vi "List Installed Packages.vi"(8 "error in":errorcluster) -> (0 "error out":errorcluster, 2 "installed packages":string[][](table))   [LabVIEW 2014, in "NIPM_API.lvlib"]
doc: "Returns a list of all installed packages, including hidden infrastructure packages.\n\nThis list is equivalent to the list of packages in the Installed tab in NI Package Manager, with \"Settings»General»Show full version numbers and infrastructure packages\" checkbox enabled.\n\nOUTPUT(s)\n<B>Installed packages</B>: Outputs a list of installed packages"
uses:
  NIPM_API.lvlib
panel:
  out "cmd standard output":string
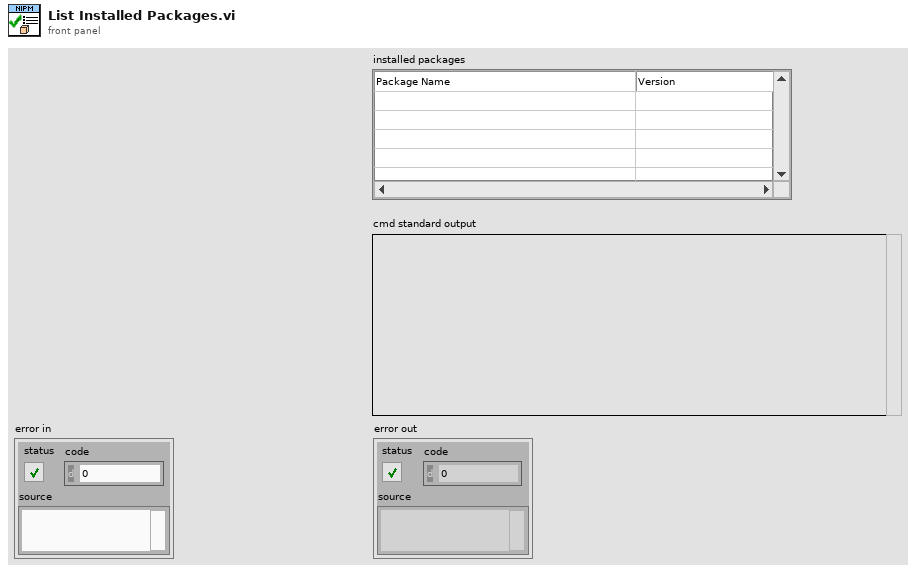
[diagram p1: front panel]
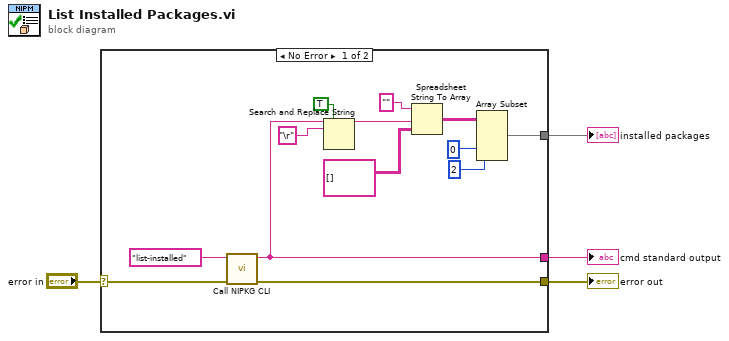
[diagram p0: block diagram]
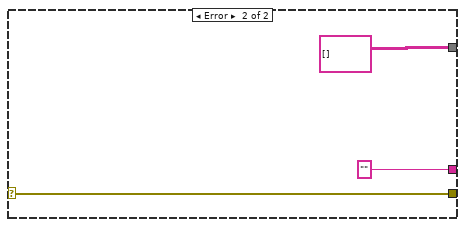
[diagram p2: hidden frame]
diagram:
  n1 = case shown="No Error" "error in" {
    selector: "error in" -> [w8 w20]
    tunnel: [w11 "" ("standard output")] -> w3
    tunnel: [w10 w20] -> w2
    tunnel: [w5 string[][] []] -> w1
    frame No Error {
      n2 = call "Call NIPKG CLI.vi"("error in (no error)"=w8, "command"="list-installed" ("format string")) -> ("error out"=w10:errorcluster, "command line standard output"=w11:string)  [unwired: 8 in]
      n3 = Search and Replace String(replace all?=TRUE ("replace all? (F)"), input string=w11, search string="\r") -> (result string=w15:string)  [unwired: 5 in, 3 out]
      n4 = Spreadsheet String To Array(format string="", spreadsheet string=w15, array type (2D Dbl)=string[][] []) -> (array=w12:string[][])  [unwired: 1 in]
      n5 = Array Subset(array=w12, index (col)=0 ("disabled index (col)"), length (col)=2 ("length")) -> (w5:string[][])  [unwired: 2 in]
    }
    frame Error {
    }
  }
  "error out" <- w2
  "cmd standard output" <- w3
  "installed packages" <- w1
